vi "Intake_Disc_Globals.vi"() -> ()   [LabVIEW 2018]
uses:
  Subsytems/Intake_Disc/Intake_Disc_Notifier.ctl
  Subsytems/Intake_Disc/Intake_Disc_Control_Type.ctl
panel:
  in  "Press_Pnuematic":string="Press_Pnuematic"
  out "Previous_Mode":bool
  out "Disc_Intaken":bool
  out "Cargo_Mode":bool
  in  "Intake_Disc_Execute_Ref":refnum<notifier>
  in  "Intake_Disc_Set_Ref":refnum<notifier>
  in  "Intake_Disc_Execute_Notifier":string="Intake_Disc_Execute_Notifier"
  in  "Intake_Disc_Set_Notifier":string="Intake_Disc_Set_Notifier"
  in  "L_Pnuematic":string="L_Pnuematic"
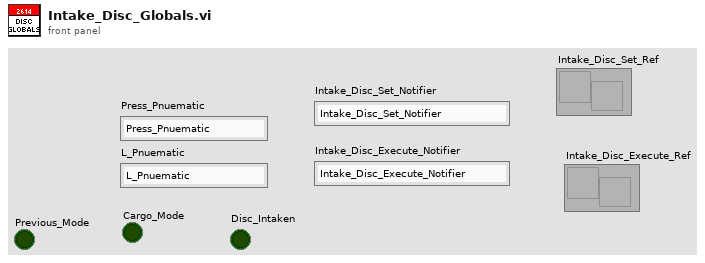
[diagram p1: front panel]
diagram:
